vi "语音播报.vi"(8 "错误输入（无错误）":errorcluster, 11 "textToSpeak":string) -> (0 "错误输出":errorcluster)   [LabVIEW 2018]
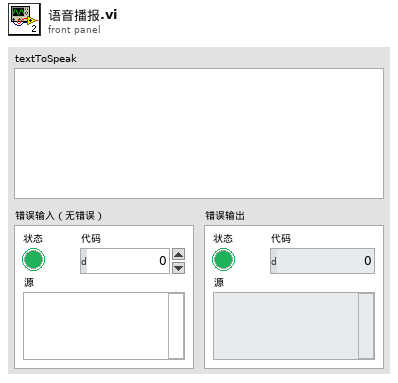
[diagram p1: front panel]
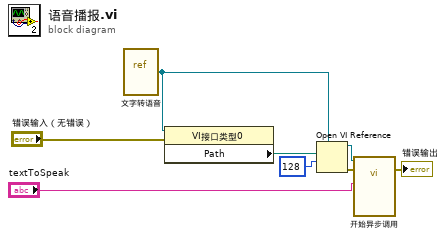
[diagram p0: block diagram]
diagram:
  n1 = vi-ref "文字转语音.vi"() -> (w5:refnum<vi>)
  n2 = property class="VI接口类型0"(reference=w5, error in="错误输入（无错误）") -> ("Path"=w6:path)  [unwired: 2 out]
  n3 = Open VI Reference(type specifier VI Refnum (for type only)=w5, vi path=w6, options=128 ("选项")) -> (vi reference=w7:refnum<vi>, error out=w2:errorcluster)  [unwired: 3 in]
  n4 = call-by-ref "开始异步调用"(reference=w7, error in=w2, "textToSpeak"="textToSpeak") -> (error out=→"错误输出":errorcluster)  [unwired: 10 in, 2 out]
